vi "Set InvWfmsQRef.vi"(8 "error in (no error)":errorcluster, 10 "InverterWaveformsQ":T1, 11 "Main in":refnum<class "Main.lvclass">) -> (0 "error out":errorcluster, 3 "Main out":refnum<class "Main.lvclass">)   [LabVIEW 2019, in "Main.lvclass"]
doc: "Developed by Kevin Thompson\nkevin@thompsonengineering.net\n\nCopyright 2018\nThompson Engineering, LLC"
uses:
  Main.lvclass
  Common/DataTypes/ChannelWaveforms--cluster.ctl
  Common/DataTypes/InverterWaveforms--cluster.ctl
  Common/DataTypes/InverterWaveforms--QRef.ctl
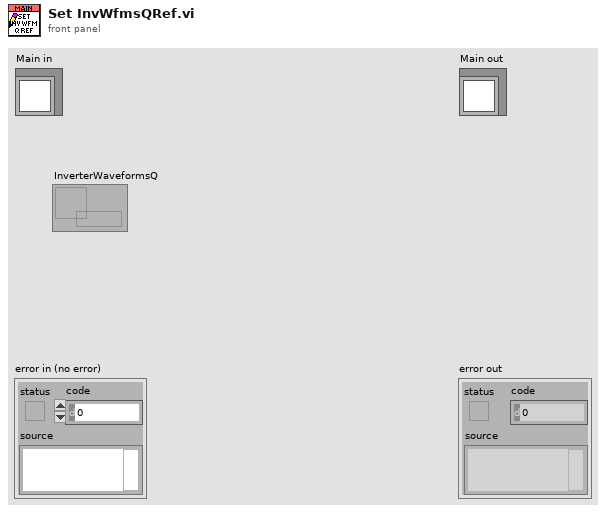
[diagram p1: front panel]
types:
  T1 = typedef "InverterWaveforms--QRef.ctl" = refnum<queue>
  T2 = typedef "Main.lvclass/ObjData--cluster.ctl" = cluster{"Settings":T3, "Public Events":T6, "Dependency":T7, "ReadData-placeholder":T8, "VISA-placeholder":refnum<visa-resource-name>, "InverterWaveformsQ":T1, "Application.TerminateProcess Event":refnum<user-event>, "RawDaqDataQ":T9, "MeasSettings":T10, "InverterDataAcqMode":T12, "DAQState Data":T13, "Private Events":T15, "InvWfmsQ-DT":T1, "DPAuxDataQ":T16, "ProcessingState":T17, "InverterInfo":T18, "CurrInverter":T19, "InverterLUT Dict":T23, "ESR Chart Ref":refnum<vi>, "StoreESR BLine Ref":refnum<vi>, "UseSavedESR BLine Ref":refnum<vi>}
  T3 = typedef "Main.lvclass/Settings--cluster.ctl" = cluster{"Simulation":bool, "Signal scaling":T4, "ESR scaling":T5, "num readings to average":i32, "ESR alarm threshhold (%)":dbl, "UseDummyVrms":bool, "Dummy Vrms":dbl, "Inverter Database File":path, "default Inverter (name)":string}
  T4 = typedef "Main.lvclass/Gain control.ctl" = cluster{"ch0 gain ":dbl, "ch1 gain":dbl, "ch2 gain ":dbl, "ch3 gain ":dbl, "ch0 offest":dbl, "ch1 offset":dbl, "ch2 offset":dbl, "ch3 offset":dbl}
  T5 = typedef "Main.lvclass/ESR scaling--cluster.ctl" = cluster{"Gain":dbl, "Offset":dbl}
  T6 = typedef "Main.lvclass/Public Events--cluster.ctl" = cluster{"Main.AsyncCmd Event":refnum<user-event>, "Main.AsyncMsg Event":refnum<user-event>, "stop process":refnum<user-event>, "UpdateControlValue Ev":refnum<user-event>, "ProcessingStateChg Ev":refnum<user-event>}
  T7 = typedef "Main.lvclass/Dependency--cluster.ctl" = cluster{"Config":refnum<class "Config.lvclass">, "DAQ":refnum<class "DAQ_Engine.lvclass">, "Log_Engine":refnum<class "Log_Engine.lvclass">}
  T8 = typedef "Main.lvclass/Read Data--cluster.ctl" = cluster{"Data":dbl}
  T9 = typedef "RawDAQDataQRef--cluster.ctl" = refnum<queue>
  T10 = typedef "Measurement Config--cluster.ctl" = cluster{"Data Rate 9775":T11, "Data Rate 9215":u32, "Samples RMS 9215":u32, "Samples RMS 9775":u32}
  T11 = typedef "nicrio_cRIO-9775_ContinuousDataRates4ChansRing.ctl" = u16
  T12 = typedef "Acquisition Mode--cluster.ctl" = enum16{"3phase", "Single"}
  T13 = typedef "DAQ_Engine.lvclass/DAQStateEvData--cluster.ctl" = cluster{"DAQState":T14, "vData":variant}
  T14 = typedef "DAQState--enum.ctl" = enum16{"Unknown", "Stopped", "Running", "Error"}
  T15 = typedef "Main.lvclass/Private Events--cluster.ctl" = cluster{"PrivateAsync Ev":refnum<user-event>}
  T16 = typedef "DataProcAuxDat--Qref.ctl" = refnum<queue>
  T17 = typedef "Main.lvclass/ProcessingState--enum.ctl" = enum16{"Idle", "Starting", "Running", "Done", "Error"}
  T18 = typedef "InverterInfo--cluster.ctl" = cluster{"Inverter ID":string}
  T19 = typedef "Inverter database record v2--cluster.ctl" = cluster{"name":string, "last updated":timestamp, "type":string, "inverter Info":T20, "gain range":T21, "offset range":T22, "gain actual":dbl, "offset actual":dbl, "power level":dbl, "minimum current":dbl, "resistance single phase":dbl, "resistance 3 phase":dbl, "set flag":u16}
  T20 = typedef "inverter info v2--cluster.ctl" = cluster{"manufacturer":string, "model":string, "product":string, "serial":string, "power class":string, "year manf":string}
  T21 = typedef "inverter gain range--cluster.ctl" = cluster{"gain max":dbl, "gain min":dbl, "gain increment":dbl}
  T22 = typedef "inverter offset range--cluster.ctl" = cluster{"offset max":dbl, "offset min":dbl, "offset increment":dbl}
  T23 = typedef "TD Dynamic CVT DVR--ref.ctl" = refnum<data-value>
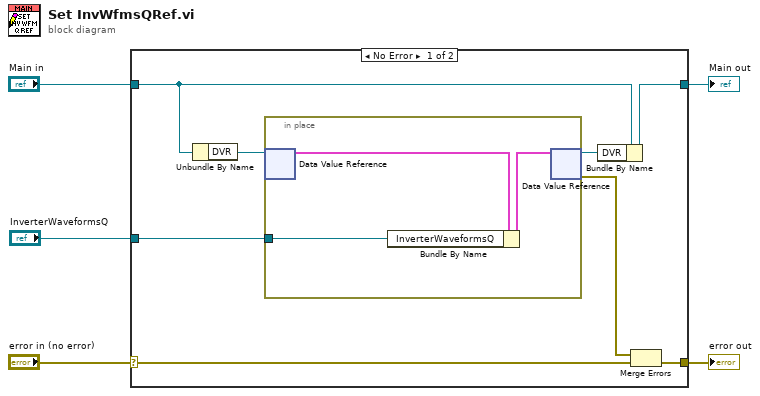
[diagram p0: block diagram]
diagram:
  n1 = case shown="No Error" "error in (no error)" {
    selector: "error in (no error)" -> [w13 w17]
    tunnel: [w7 w17] -> w4
    tunnel: [w9 w18] -> w2
    tunnel: "Main in" -> [w12 w18]
    tunnel: "InverterWaveformsQ" -> [w8 _]
    frame No Error {
      n2 = Unbundle By Name(w12) -> ("DVR"=w11:refnum<data-value>)
      n3 = in-place {
        in-place-border: w8 -> [w14]
        n4 = in-place-dvr #1(w11) -> (w16:T2)  [unwired: 1 out]
        n5 = Bundle By Name(cluster=w16, "InverterWaveformsQ"=w14) -> (w15:T2)
        n6 = in-place-dvr #1(w15) -> (w10:refnum<data-value>, w6:errorcluster)
      }
      n7 = Bundle By Name(cluster=w12, "DVR"=w10) -> (w9:refnum<class "Main.lvclass">)
      n8 = Merge Errors(w6, w13) -> (w7:errorcluster)
    }
    frame Error {
    }
  }
  "error out" <- w4
  "Main out" <- w2
